vi "Configure MCCW Carriers.vi"(8 "error in (no error)":errorcluster, 9 "MCCW Carrier spacing [Hz]":dbl, 10 "MCCW Carriers":i32, 11 "VSG-SMBV in":refnum<class "VSG-SMBV.lvclass">) -> (0 "error out":errorcluster, 3 "VSG-SMBV out":refnum<class "VSG-SMBV.lvclass">)   [LabVIEW 2020, in "VSG-SMBV.lvclass"]
doc: "Configure the number and spacing for carriers in the MCCW."
uses:
  VSG-SMBV.lvclass
  C:/Sandbox/Git_Sandbox/WiSpry Test Framework source code (LV20)/WiSpry Test Framework/Instruments/Instrument.lvclass
  Instrument.lvclass/Instrument.ctl
  Instrument.lvclass
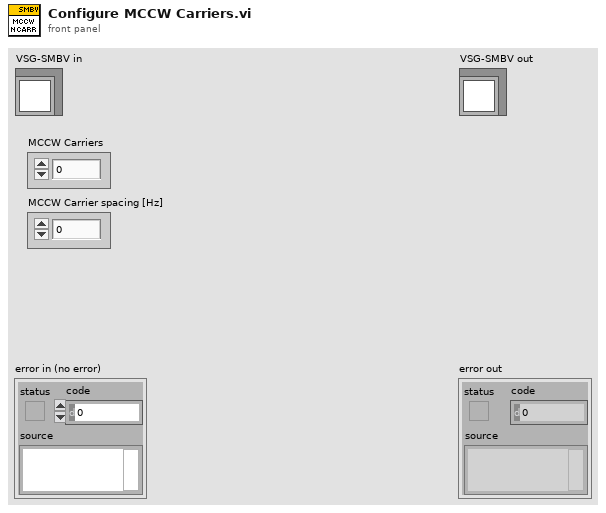
[diagram p1: front panel]
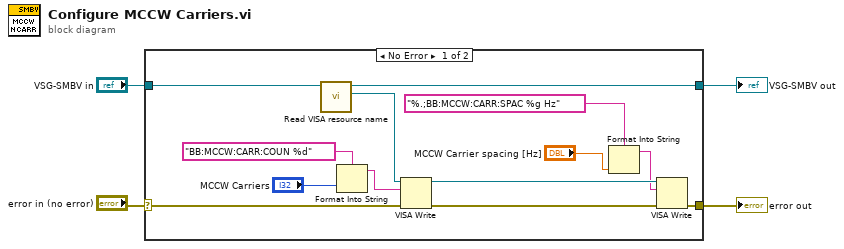
[diagram p0: block diagram]
diagram:
  n1 = case shown="No Error" "error in (no error)" {
    selector: "error in (no error)" -> [w15 w18]
    tunnel: "VSG-SMBV in" -> [w17 w19]
    tunnel: [w9 w18] -> w2
    tunnel: [w5 w19] -> w1
    frame No Error {
      n2 = call "Read VISA resource name.vi"("Instrument in"=w17) -> ("VISA resource name"=w16:refnum<visa-resource-name>, "Instrument out"=w5:refnum<class "VSG-SMBV.lvclass">)  [unwired: 9 in]
      n3 = Format Into String(format string="BB:MCCW:CARR:COUN %d", "MCCW Carriers") -> (resulting string=w12:string)  [unwired: 2 in, 1 out]
      n4 = VISA Write(VISA resource name=w16, write buffer=w12, error in (no error)=w15) -> (VISA resource name out=w8:refnum<visa-resource-name>, error out=w7:errorcluster)  [unwired: 1 out]
      n5 = Format Into String(format string="%.;BB:MCCW:CARR:SPAC %g Hz", "MCCW Carrier spacing [Hz]") -> (resulting string=w6:string)  [unwired: 2 in, 1 out]
      n6 = VISA Write(VISA resource name=w8, write buffer=w6, error in (no error)=w7) -> (error out=w9:errorcluster)  [unwired: 2 out]
    }
    frame Error {
    }
  }
  "error out" <- w2
  "VSG-SMBV out" <- w1
